vi "Run Timing Test.vi"(7 "Number of Concurrent Calls (4)":i32=4, 8 "error in (no error)":errorcluster, 9 "Number of Iterations (12000)":i32=12000, 10 "Period (msec)":i64=10, 11 "address":string="localhost:50051") -> (0 "error out":errorcluster, 2 "Timing Stats":T1, 3 "All Roundtrip Measurments (usec)":string)   [LabVIEW 2021]
uses:
  TYPEDEF - Timing Statistics.ctl
  TYPEDEF - Timing Statistics with Iteration Number.ctl
  <vilib>/Platform/TimedLoop/XDataNode/timing_clust.ctl
  <vilib>/Platform/TimedLoop/XDataNode/nitl_modes.ctl
  <vilib>/Platform/TimedLoop/XDataNode/wakeup.ctl
  <vilib>/platform/TimedLoop/XDataNode/XDataNode.xnode
  <vilib>/Platform/TimedLoop/XDataNode/XDNodeRunTimeDep.lvlib
  gRPC/test_service_client/test_service_client.lvlib
  <vilib>/Analysis/NI_AALBase.lvlib
  TYPEDEF - Overall Timing Statistics.ctl
panel:
  out "Current Roundtrip Call Duration (usec)":u64
  out "Long Calls (1000+ usec)":T2[](array[typedef])
  out "Number of Long Calls":i32
  out "Longest Statistic":T3
  out "Iteration":i32
  in  "stop":bool
  # "^^^Can be used to put into Excel\nafter this VI runs"
  # "^^^ Shows on the fly reporting of long roundtrip measurements (1000+ usec)"
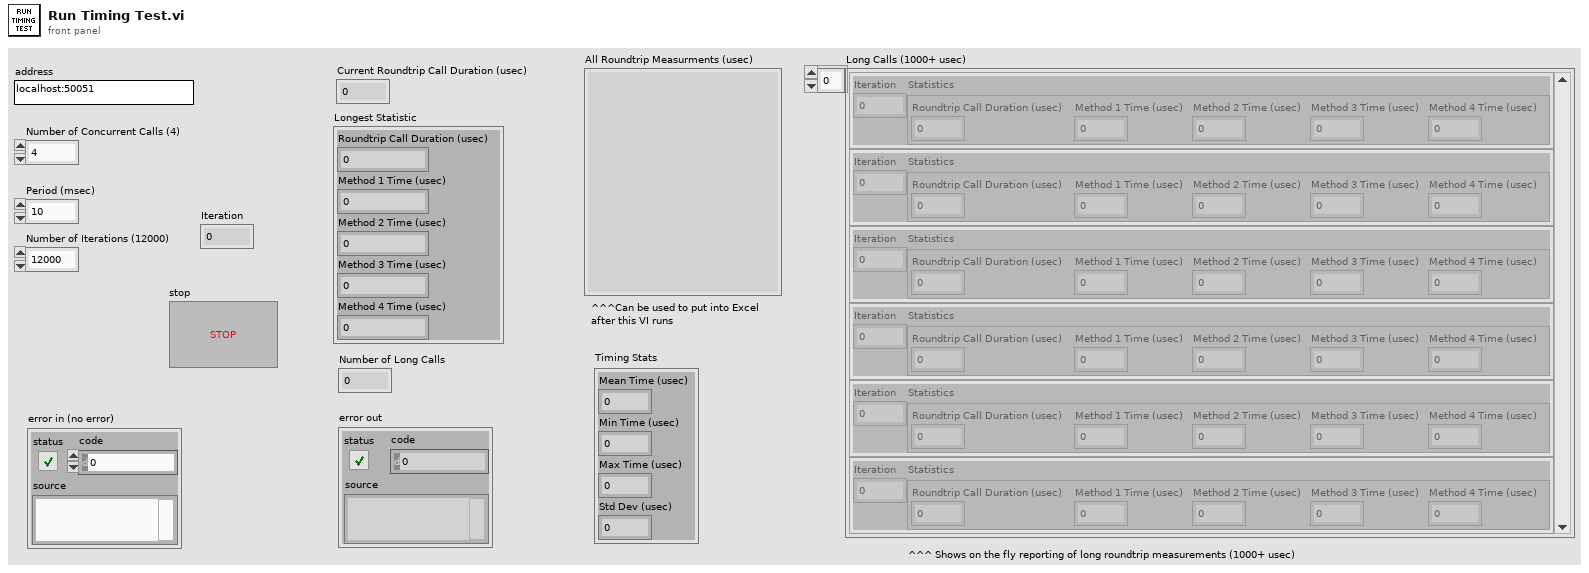
[diagram p1: front panel]
types:
  T1 = typedef "TYPEDEF - Overall Timing Statistics.ctl" = cluster{"Mean Time (usec)":dbl, "Min Time (usec)":dbl, "Max Time (usec)":dbl, "Std Dev (usec)":dbl}
  T2 = typedef "TYPEDEF - Timing Statistics with Iteration Number.ctl" = cluster{"Iteration":i32, "Statistics":T3}
  T3 = typedef "TYPEDEF - Timing Statistics.ctl" = cluster{"Roundtrip Call Duration (usec)":u64, "Method 1 Time (usec)":u64, "Method 2 Time (usec)":u64, "Method 3 Time (usec)":u64, "Method 4 Time (usec)":u64}
  T4 = typedef "XDNodeRunTimeDep.lvlib/timing_clust.ctl" = cluster{"Expected End [f-1]":u64, "Actual End [f-1]":u64, "Finished Late? [f-1]":bool, "Expected End [i-1]":u64, "Actual End [i-1]":u64, "Finished Late? [i-1]":bool, "Expected Start [i]":u64, "Actual Start [i]":u64, "Expected Start [f]":u64, "Actual Start [f]":u64, "Source Name":string, "Structure Name":string, "Period":i64, "Deadline":i64, "Offset":i64, "Start":i64, "Priority":i32, "Timeout":i32, "Mode":T5, "Wakeup Reason":T6, "Error":errorcluster, "Source Type":string, "Secondary Source Type":string, "Global End Time":u64, "Global Start Time":u64, "Frame Duration":u64, "Iteration Duration":u64, "Assigned CPU":i32, "I/O Scan Engine Mode":u32}
  T5 = typedef "XDNodeRunTimeDep.lvlib/nitl_modes.ctl" = enum32{"No Change", "Process missed periods, maintain original phase", "Discard missed periods, maintain original phase", "Process missed periods, ignore original phase", "Discard missed periods, ignore original phase"}
  T6 = typedef "XDNodeRunTimeDep.lvlib/wakeup.ctl" = enum32{"Normal", "Aborted", "Asynchronous wakeup", "Timing source error", "Timed loop error", "Timeout"}
  T7 = typedef "grpc-lvsupport-release.lvlib/grpcId.ctl" = u64
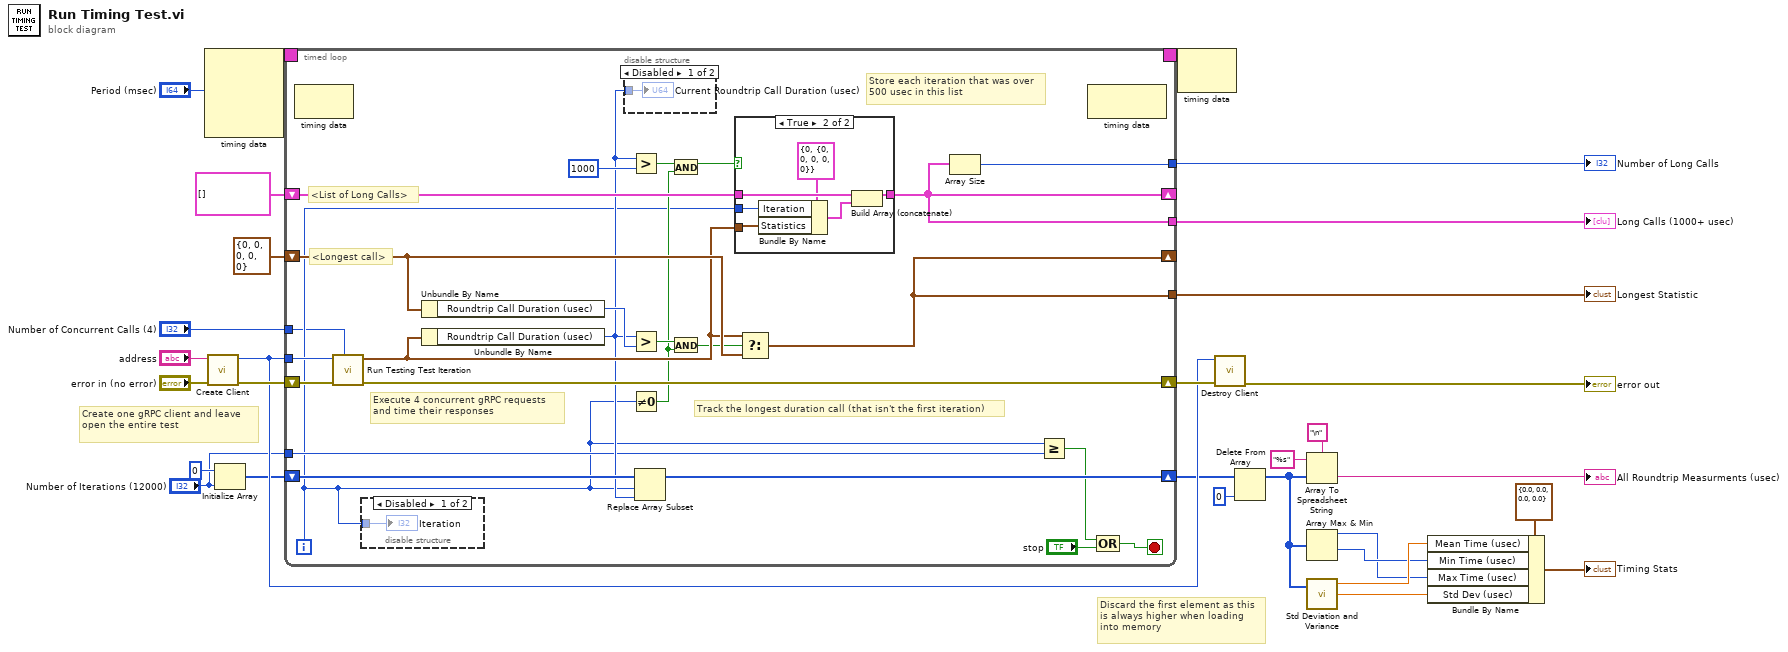
[diagram p0: block diagram]
diagram:
  # "Discard the first element as this\nis always higher when loading\ninto memory"
  # "Create one gRPC client and leave open the entire test"
  n1 = node-c288("Period (msec)") -> (w30:T4)  [unwired: 3 in]
  n2 = call "Create Client.vi"("error in"="error in (no error)", "address"="address") -> ("error out"=w27:errorcluster, "gRPC ID Out"=w25:T7)  [unwired: 8 in]
  n3 = Initialize Array(u64 0 ("element"), "Number of Iterations (12000)") -> (w18:u64[])
  n4 = timed-loop {
    timing: w30 -> [_]
    timing-out: [_] -> w29
    tunnel: w25 -> [w55]
    shift-right: [w53] -> w26
    shift-left: w27 -> [w54]
    shift-right: [w33] -> _
    shift-left: T3 {"Roundtrip Call Duration (usec)"=0, "Method 1 Time (usec)"=0, "Method 2 Time (usec)"=0, "Method 3 Time (usec)"=0, "Method 4 Time (usec)"=0} ("Timing Statistics") -> [w50]
    shift-right: [w32] -> _
    shift-left: T2[] [] -> [w48]
    shift-right: [w43] -> w9
    shift-left: w18 -> [w44]
    tunnel: "Number of Iterations (12000)" -> [w40]
    tunnel: "Number of Concurrent Calls (4)" -> [w34]
    tunnel: [w33] -> w12
    tunnel: [w32] -> w11
    tunnel: [w31] -> w10
    i -> [w35]
    stop <- w42 stop-if-true
    # "Store each iteration that was over\n500 usec in this list"
    # "Track the longest duration call (that isn't the first iteration)"
    # "Execute 4 concurrent gRPC requests\nand time their responses"
    # "<List of Long Calls>"
    # "<Longest call>"
    n5 = node-c288() -> ()  [unwired: 1 in, 1 out]
    n6 = call "Run Testing Test Iteration.vi"("Number of Concurrent Calls (4)"=w34, "error in (no error)"=w54, "gRPC ID"=w55) -> ("error out"=w53:errorcluster, "Timing Statistics"=w47:T3)  [unwired: 7 in]
    n7 = disable-structure shown="Disabled" {
      disable-tunnel: w35 -> [w57 _]
      frame Disabled {
        "Iteration" <- w57
      }
      frame Enabled {
      }
    }
    n8 = Unbundle By Name(w50) -> ("Roundtrip Call Duration (usec)"=w51:u64)
    n9 = Unbundle By Name(w47) -> ("Roundtrip Call Duration (usec)"=w41:u64)
    n10 = disable-structure shown="Disabled" {
      disable-tunnel: w41 -> [w56 _]
      frame Disabled {
        "Current Roundtrip Call Duration (usec)" <- w56
      }
      frame Enabled {
      }
    }
    n11 = Greater?(x=w41, y=u64 1000) -> (0:w38:bool)
    n12 = Greater?(x=w41, y=w51) -> (0:w46:bool)
    n13 = Not Equal To 0?(x=w35) -> (x != 0?=w37:bool)
    n14 = Replace Array Subset(array=w44, new element=w41, index=w35) -> (w43:u64[])
    n15 = And(x=w38, y=w37) -> (x .and. y?=w36:bool)
    n16 = And(x=w46, y=w37) -> (x .and. y?=w45:bool)
    n17 = case shown="True" w36 {
      tunnel: w48 -> [w58 w64]
      tunnel: w47 -> [_ w61]
      tunnel: [w58 w63] -> w32
      tunnel: w35 -> [_ w60]
      frame False {
      }
      frame True {
        n18 = Bundle By Name(cluster=T2 {"Iteration"=0, "Statistics"={"Roundtrip Call Duration (usec)"=0, "Method 1 Time (usec)"=0, "Method 2 Time (usec)"=0, "Method 3 Time (usec)"=0, "Method 4 Time (usec)"=0}}, "Iteration"=w60, "Statistics"=w61) -> (w59:T2)
        n19 = Build Array (concatenate)(w64, w59) -> (w63:T2[])
      }
    }
    n20 = Select(t=w47, s=w45, f=w50) -> (s? t:f=w33:T3)
    n21 = Array Size(array=w32) -> (size(s)=w31:i32)
    n22 = Greater Or Equal?(x=w35, y=w40) -> (x >= y?=w39:bool)
    n23 = node-c288() -> ()  [unwired: 1 in, 1 out]
    n24 = Compound Arithmetic op=OR(w39, "stop") -> (w42:bool)
  }
  "Longest Statistic" <- w12
  "Number of Long Calls" <- w10
  "Long Calls (1000+ usec)" <- w11
  n25 = node-c288(w29) -> ()  [unwired: 1 out]
  n26 = call "Destroy Client.vi"("error in"=w26, "gRPC ID"=w25) -> ("error out"=→"error out":errorcluster)  [unwired: 9 in]
  n27 = Delete From Array(array=w9, index=0) -> (array with subset deleted=w1:u64[])  [unwired: 1 in, 1 out]
  n28 = Array To Spreadsheet String(delimiter (Tab)="\n", array=w1, 3:"%s" ("format string")) -> (spreadsheet string=→"All Roundtrip Measurments (usec)":string)
  n29 = Array Max & Min(array=w1) -> (max value=w3:u64, min value=w4:u64)  [unwired: 2 out]
  n30 = call <vilib>:"Std Deviation and Variance.vi"("X"=w1) -> ("mean"=w5:dbl, "standard deviation"=w6:dbl)  [unwired: 1 in, 1 out]
  n31 = Bundle By Name(cluster=T1 {"Mean Time (usec)"=0.0, "Min Time (usec)"=0.0, "Max Time (usec)"=0.0, "Std Dev (usec)"=0.0} ("Timing Stats"), "Mean Time (usec)"=w5, "Min Time (usec)"=w4, "Max Time (usec)"=w3, "Std Dev (usec)"=w6) -> (→"Timing Stats":T1)
